vi "mbed.vi"() -> (0 "Array of Numbers":dbl[](array[numeric]), 2 "Array of Strings":string[](array[string]), 3 "Line String":string)   [LabVIEW 2009]
uses:
  <vilib>/Instr/_visa.llb/VISA Configure Serial Port (Instr).vi
panel:
  out "Status":errorcluster
  out "VISA resource name out":refnum<visa-resource-name>
  in  "Baud Rate":u32=9600
  in  "Serial Port":refnum<visa-resource-name>
  # "mbed Serial Settings"
  # "Output Data"
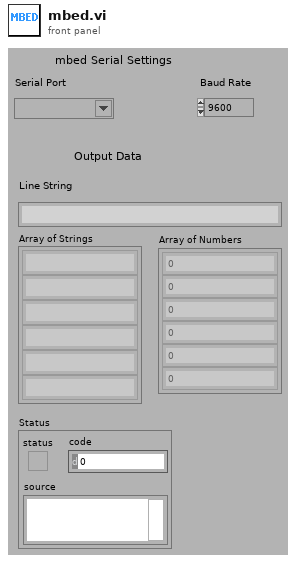
[diagram p1: front panel]
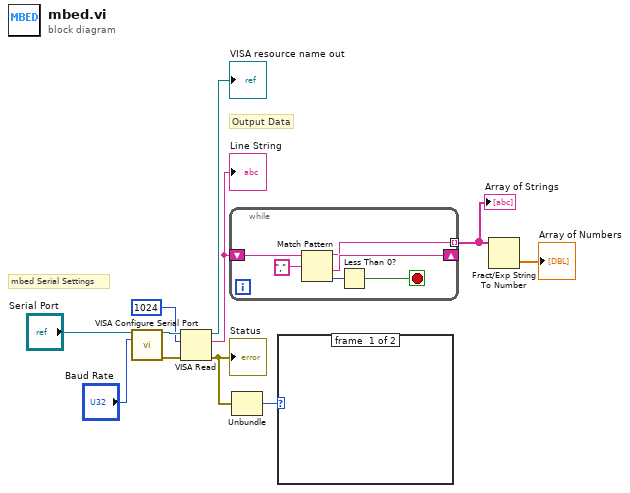
[diagram p0: block diagram]
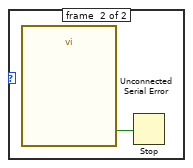
[diagram p2: hidden frame]
diagram:
  # "Output Data"
  # "mbed Serial Settings"
  n1 = call-poly "VISA Configure Serial Port"("VISA resource name"="Serial Port", "baud rate (9600)"="Baud Rate") -> ("VISA resource name out"=w9:refnum<visa-resource-name>, "error out"=w8:errorcluster)  [unwired: 12 in]
  n2 = VISA Read(VISA resource name=w9, byte count=u32 1024, error in (no error)=w8) -> (VISA resource name out=→"VISA resource name out":refnum<visa-resource-name>, read buffer=w4:string, error out=w2:errorcluster)  [unwired: 1 out]
  "Line String" <- w4
  "Status" <- w2
  n3 = while {
    tunnel: [w14] -> w5 mode=indexing
    shift-right: [w15] -> _
    shift-left: w4 -> [w17]
    stop <- w12 stop-if-true
    n4 = Match Pattern(string=w17, regular expression=",") -> (before substring=w14:string, after substring=w15:string, offset past match=w13:i32)  [unwired: 2 out]
    n5 = Less Than 0?(x=w13) -> (x < 0?=w12:bool)
  }
  "Array of Strings" <- w5
  n6 = Unbundle(w2) -> ("code"=w1:i32)  [unwired: 2 out]
  n7 = case shown="1" w1 {
    frame #0 {
    }
    frame #1 {
      n8 = call "Unconnected Serial Error"() -> ("OK"=w18:bool)  [unwired: 10 in, 1 out]
      n9 = Stop(stop? (T)=w18) -> ()
    }
  }
  n10 = Fract/Exp String To Number(string=w5) -> (number=→"Array of Numbers":dbl[])  [unwired: 3 in, 1 out]
